vi "Close.vi"(8 "error in (no error)":errorcluster, 11 "HttpContent in":refnum<class "HttpContent.lvclass">) -> (0 "error out":errorcluster)   [LabVIEW 2018, in "HttpClient_NET.lvlib" / "HttpContent.lvclass"]
uses:
  HttpContent.lvclass
  HttpContent.lvclass/HttpContent.ctl
  System.Net.Http
  Accessors/Read NET_HttpContent.vi
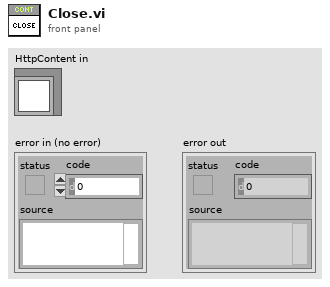
[diagram p1: front panel]
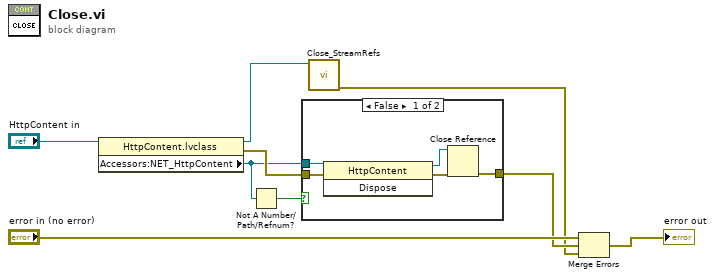
[diagram p0: block diagram]
diagram:
  n1 = property class="HttpContent.lvclass"(reference="HttpContent in") -> (reference out=w2:refnum<class "HttpContent.lvclass">, error out=w7:errorcluster, "Accessors:NET_HttpContent"=w4:refnum<k24>)  [unwired: 1 in]
  n2 = Not A Number/Path/Refnum?(number/path/refnum=w4) -> (NaN/Path/Refnum?=w3:bool)
  n3 = case shown="False" w3 {
    tunnel: w7 -> [w12 w15]
    tunnel: [w11 w15] -> w5
    tunnel: w4 -> [w10 _]
    frame False {
      n4 = invoke class="HttpContent" method="Dispose"(reference=w10, error in=w12) -> (reference out=w13:refnum<k24>, error out=w14:errorcluster)  [unwired: 1 in, 1 out]
      n5 = Close Reference(reference=w13, error in (no error)=w14) -> (error out=w11:errorcluster)
    }
    frame True {
    }
  }
  n6 = call "Close_StreamRefs.vi"("HttpContent in"=w2) -> ("error out"=w1:errorcluster)  [unwired: 9 in, 1 out]
  n7 = Merge Errors("error in (no error)", w5, w1) -> (→"error out":errorcluster)
